vi "Format Script Email.vi"(8 "Script Start/End":enum16{"Start Script", "End Script"}(ring), 9 "Time String":string, 11 "Measurement Information":T1={"Comments"="", "Directory Input"="", "Data file path"=path "C:/Data/EPR Data", "Scripting File"=path "C:/Data/Configuration Script.csv", "Save Data"=FALSE, "Tooth size (d11) [mm]"=0.0, "Tooth size (d12) [mm]"=0.0, "Tooth size (d21) [mm]"=0.0, "Tooth size (d22) [mm]"=0.0, "Dose of Tooth [Gy]"=0.0, "Safe Shutdown?"=FALSE, "Gases Available"=[], "Database Username"="", "Database Password"="", "Database Login URL"="", "Database Upload URL"="", "Database Success URL"="", "Database XML URL"="", "Database Resonator URL"="", "Session Number"=0, "Set #"=0, "Resonator Operator"="", "Session Type"="", "Tooth/Sample ID"="", "Volunteer ID"="", "Computer Operator"="", "Volunteer Type"="", "Site/Tooth Selection (T8,T9)"="", "Resonator"="", "Measurement Site"="", "Non-standard session?"=FALSE, "EPR DAQ Version"="", "Session Path"=path "C:/Data/EPR Data", "Chosen Applied State"="", "Chosen Initial State"="", "Time of Transition"="", "DAQ Mode"=enum."Engineering", "pO2/Scan [mmHg]"=[], "pO2/Set [mmHg]"=[], "Linewidth (HWHM)/Scan [Gauss]"=[], "Linewidth (HWHM)/Set [Gauss]"=[], "pO2 Conversion"="", "Dose Calibration Cluster"={"Dose Response"={"grand_mean"=0.0292016, "slope"=0.0188720543}, "Dose Correction"={"Sex"=1, "a0"=7.719669421, "a1"=-2.746550736, "a2"=-0.186490355, "a3"=0.041922063, "a4"=-0.849147359, "a5"=0.14330063, "a6"=0.019930219, "A_n"=40.0, "H_n"=10.12, "Dose Correction"=FALSE}, "Dose Reporting"={"Reporting is"=TRUE, "sd_threshold [AU]"=0.06, "sd_model [Gy]"=0.66, "dosimetric_threshold [Gy]"=2.0, "Add intrasession errors is"=FALSE, "Prior Radiation?"=FALSE}}, "OxyChip Slope"=0.0, "OxyChip Intercept"=0.0, "QA Mode"=enum."Select QA Mode", "QA Session?"=FALSE, "Sample Type"=enum."Empty Resonator", "Report pO2/Scan"=FALSE, "Skip End Session Save"=FALSE, "Number of sites"=enum."# Probes", "Recipient Name"="", "Sender Name"="", "Recipient Email"="", "Transition State History"=[], "pO2 Report Times"=[], "Temperature [C]"=0.0, "+Error pO2/Scan [mmHg]"=[], "-Error pO2/Scan [mmHg]"=[], "+Error pO2/Set [mmHg]"=[], "-Error pO2/Set [mmHg]"=[], "Oxy Phase Exclusion Tolerance [rad]"=0.0, "Oxy Center Exclusion Tolerance [%]"=0.0, "Oxy Exclude Unacceptable"=FALSE, "Oxy Unacceptable Estimate Flags"=[], "Save Session PPT"=FALSE, "Flagged Bad Sets"=[]} {"Oxy Center Exclusion Tolerance [%]" format="%#_9g"; "Oxy Phase Exclusion Tolerance [rad]" format="%#_9g"; "Temperature [C]" format="%#_9g"; "OxyChip Intercept" format="%#_9g"; "OxyChip Slope" format="%#_9g"; "Dose Calibration Cluster"."Dose Reporting"."dosimetric_threshold [Gy]" format="%#_9g"; "Dose Calibration Cluster"."Dose Reporting"."sd_model [Gy]" format="%#_9g"; "Dose Calibration Cluster"."Dose Reporting"."sd_threshold [AU]" format="%#_9g"; "Dose Calibration Cluster"."Dose Correction"."H_n" format="%#_9g"; "Dose Calibration Cluster"."Dose Correction"."A_n" format="%#_9g"; "Dose Calibration Cluster"."Dose Correction"."a6" format="%#.9g"; "Dose Calibration Cluster"."Dose Correction"."a5" format="%#.9g"; "Dose Calibration Cluster"."Dose Correction"."a4" format="%#.9g"; "Dose Calibration Cluster"."Dose Correction"."a3" format="%#.9g"; "Dose Calibration Cluster"."Dose Correction"."a2" format="%#.9g"; "Dose Calibration Cluster"."Dose Correction"."a1" format="%#.9g"; "Dose Calibration Cluster"."Dose Correction"."a0" format="%#.9g"; "Dose Calibration Cluster"."Dose Correction"."Sex" items=["Male"=1, "Female"=0]; "Dose Calibration Cluster"."Dose Response"."slope" format="%#_9g"; "Dose Calibration Cluster"."Dose Response"."grand_mean" format="%#_9g"}) -> (3 "Measurement Information Out":T1={"Comments"="", "Directory Input"="", "Data file path"=path "C:/Data/EPR Data", "Scripting File"=path "C:/Data/Configuration Script.csv", "Save Data"=FALSE, "Tooth size (d11) [mm]"=0.0, "Tooth size (d12) [mm]"=0.0, "Tooth size (d21) [mm]"=0.0, "Tooth size (d22) [mm]"=0.0, "Dose of Tooth [Gy]"=0.0, "Safe Shutdown?"=FALSE, "Gases Available"=[], "Database Username"="", "Database Password"="", "Database Login URL"="", "Database Upload URL"="", "Database Success URL"="", "Database XML URL"="", "Database Resonator URL"="", "Session Number"=0, "Set #"=0, "Resonator Operator"="", "Session Type"="", "Tooth/Sample ID"="", "Volunteer ID"="", "Computer Operator"="", "Volunteer Type"="", "Site/Tooth Selection (T8,T9)"="", "Resonator"="", "Measurement Site"="", "Non-standard session?"=FALSE, "EPR DAQ Version"="", "Session Path"=path "C:/Data/EPR Data", "Chosen Applied State"="", "Chosen Initial State"="", "Time of Transition"="", "DAQ Mode"=enum."Engineering", "pO2/Scan [mmHg]"=[], "pO2/Set [mmHg]"=[], "Linewidth (HWHM)/Scan [Gauss]"=[], "Linewidth (HWHM)/Set [Gauss]"=[], "pO2 Conversion"="", "Dose Calibration Cluster"={"Dose Response"={"grand_mean"=0.0292016, "slope"=0.0188720543}, "Dose Correction"={"Sex"=1, "a0"=7.719669421, "a1"=-2.746550736, "a2"=-0.186490355, "a3"=0.041922063, "a4"=-0.849147359, "a5"=0.14330063, "a6"=0.019930219, "A_n"=40.0, "H_n"=10.12, "Dose Correction"=FALSE}, "Dose Reporting"={"Reporting is"=TRUE, "sd_threshold [AU]"=0.06, "sd_model [Gy]"=0.66, "dosimetric_threshold [Gy]"=2.0, "Add intrasession errors is"=FALSE, "Prior Radiation?"=FALSE}}, "OxyChip Slope"=0.0, "OxyChip Intercept"=0.0, "QA Mode"=enum."Select QA Mode", "QA Session?"=FALSE, "Sample Type"=enum."Empty Resonator", "Report pO2/Scan"=FALSE, "Skip End Session Save"=FALSE, "Number of sites"=enum."# Probes", "Recipient Name"="", "Sender Name"="", "Recipient Email"="", "Transition State History"=[], "pO2 Report Times"=[], "Temperature [C]"=0.0, "+Error pO2/Scan [mmHg]"=[], "-Error pO2/Scan [mmHg]"=[], "+Error pO2/Set [mmHg]"=[], "-Error pO2/Set [mmHg]"=[], "Oxy Phase Exclusion Tolerance [rad]"=0.0, "Oxy Center Exclusion Tolerance [%]"=0.0, "Oxy Exclude Unacceptable"=FALSE, "Oxy Unacceptable Estimate Flags"=[], "Save Session PPT"=FALSE, "Flagged Bad Sets"=[]} {"Oxy Center Exclusion Tolerance [%]" format="%#_9g"; "Oxy Phase Exclusion Tolerance [rad]" format="%#_9g"; "Temperature [C]" format="%#_9g"; "OxyChip Intercept" format="%#_9g"; "OxyChip Slope" format="%#_9g"; "Dose Calibration Cluster"."Dose Reporting"."dosimetric_threshold [Gy]" format="%#_9g"; "Dose Calibration Cluster"."Dose Reporting"."sd_model [Gy]" format="%#_9g"; "Dose Calibration Cluster"."Dose Reporting"."sd_threshold [AU]" format="%#_9g"; "Dose Calibration Cluster"."Dose Correction"."H_n" format="%#_9g"; "Dose Calibration Cluster"."Dose Correction"."A_n" format="%#_9g"; "Dose Calibration Cluster"."Dose Correction"."a6" format="%#.9g"; "Dose Calibration Cluster"."Dose Correction"."a5" format="%#.9g"; "Dose Calibration Cluster"."Dose Correction"."a4" format="%#.9g"; "Dose Calibration Cluster"."Dose Correction"."a3" format="%#.9g"; "Dose Calibration Cluster"."Dose Correction"."a2" format="%#.9g"; "Dose Calibration Cluster"."Dose Correction"."a1" format="%#.9g"; "Dose Calibration Cluster"."Dose Correction"."a0" format="%#.9g"; "Dose Calibration Cluster"."Dose Correction"."Sex" items=["Male"=1, "Female"=0]; "Dose Calibration Cluster"."Dose Response"."slope" format="%#_9g"; "Dose Calibration Cluster"."Dose Response"."grand_mean" format="%#_9g"})   [LabVIEW 2016]
uses:
  Types/Measurement Information.ctl
  Analysis/Dose Calculation and Reporting/Dose Calculation Control.ctl
  Types/Sample Type.ctl
panel:
  in  "Cancel":bool
  in  "Continue":bool
  in  "Email Address of Recipient":string
  in  "Name of Recipient":string
  in  "Name of Sender":string
  # "Session Information"
  # "Oximetric Data and Information"
  # "Email"
  # "Tooth Information"
  # "Database"
  # "Session Information"
  # "Oximetric Data and Information"
  # "Email"
  # "Tooth Information"
  # "Database"
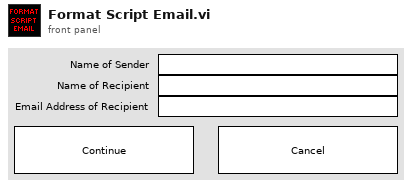
[diagram p1: front panel]
types:
  T1 = typedef "Measurement Information.ctl" = cluster{"Comments":string, "Directory Input":string, "Data file path":path, "Scripting File":path, "Save Data":bool, "Tooth size (d11) [mm]":dbl, "Tooth size (d12) [mm]":dbl, "Tooth size (d21) [mm]":dbl, "Tooth size (d22) [mm]":dbl, "Dose of Tooth [Gy]":dbl, "Safe Shutdown?":bool, "Gases Available":string[], "Database Username":string, "Database Password":string, "Database Login URL":string, "Database Upload URL":string, "Database Success URL":string, "Database XML URL":string, "Database Resonator URL":string, "Session Number":i32, "Set #":u32, "Resonator Operator":string, "Session Type":string, "Tooth/Sample ID":string, "Volunteer ID":string, "Computer Operator":string, "Volunteer Type":string, "Site/Tooth Selection (T8,T9)":string, "Resonator":string, "Measurement Site":string, "Non-standard session?":bool, "EPR DAQ Version":string, "Session Path":path, "Chosen Applied State":string, "Chosen Initial State":string, "Time of Transition":string, "DAQ Mode":enum16{"Engineering", "Dosimetry", "Oximetry"}, "pO2/Scan [mmHg]":dbl[][], "pO2/Set [mmHg]":dbl[][], "Linewidth (HWHM)/Scan [Gauss]":dbl[][], "Linewidth (HWHM)/Set [Gauss]":dbl[][], "pO2 Conversion":string, "Dose Calibration Cluster":T2, "OxyChip Slope":dbl, "OxyChip Intercept":dbl, "QA Mode":enum16{"Select QA Mode", "QA-Start/End", "QA-Mid", "QA-Weekly", "QA-Eng", "Check Calibration"}, "QA Session?":bool, "Sample Type":T3, "Report pO2/Scan":bool, "Skip End Session Save":bool, "Number of sites":enum16{"# Probes", "1", "2", "3", "4"}, "Recipient Name":string, "Sender Name":string, "Recipient Email":string, "Transition State History":string[], "pO2 Report Times":string[], "Temperature [C]":dbl, "+Error pO2/Scan [mmHg]":dbl[][], "-Error pO2/Scan [mmHg]":dbl[][], "+Error pO2/Set [mmHg]":dbl[][], "-Error pO2/Set [mmHg]":dbl[][], "Oxy Phase Exclusion Tolerance [rad]":dbl, "Oxy Center Exclusion Tolerance [%]":dbl, "Oxy Exclude Unacceptable":bool, "Oxy Unacceptable Estimate Flags":bool[], "Save Session PPT":bool, "Flagged Bad Sets":u32[]}
  T2 = typedef "Dose Calculation Control.ctl" = cluster{"Dose Response":cluster{"grand_mean":dbl, "slope":dbl}, "Dose Correction":cluster{"Sex":u16, "a0":dbl, "a1":dbl, "a2":dbl, "a3":dbl, "a4":dbl, "a5":dbl, "a6":dbl, "A_n":dbl, "H_n":dbl, "Dose Correction":bool}, "Dose Reporting":cluster{"Reporting is":bool, "sd_threshold [AU]":dbl, "sd_model [Gy]":dbl, "dosimetric_threshold [Gy]":dbl, "Add intrasession errors is":bool, "Prior Radiation?":bool}}
  T3 = typedef "Sample Type.ctl" = enum16{"Empty Resonator", "IRS", "BallZero", "Irradiated Tooth", "Non-irradiated Tooth", "OxyChip", "LiPc", "PDT", "India Ink"}
  T4 = enum8{"Enabled", "Disabled", "Disabled and Grayed Out"}
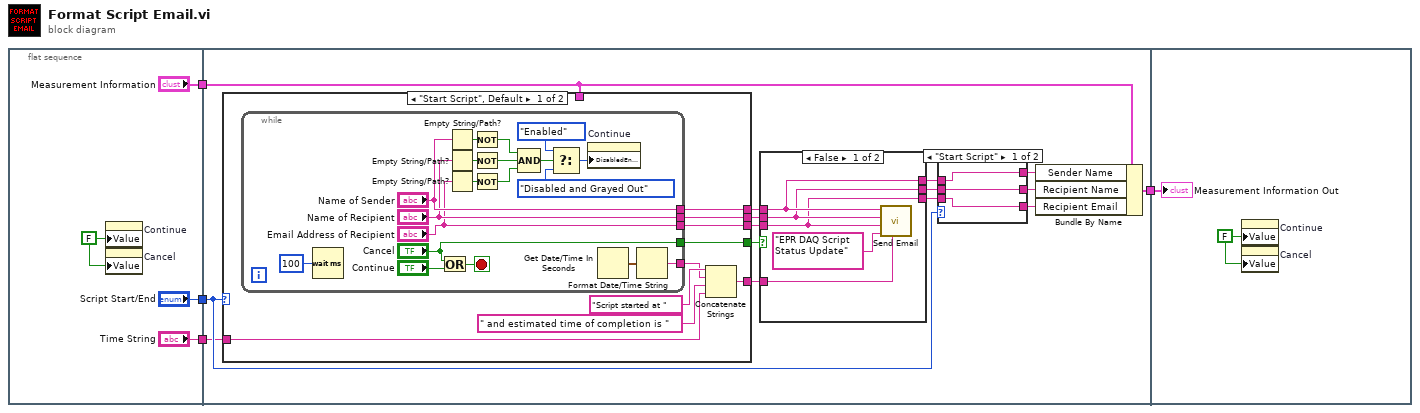
[diagram p0: block diagram]
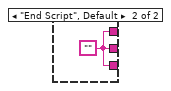
[diagram p2: hidden frame]
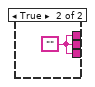
[diagram p3: hidden frame]
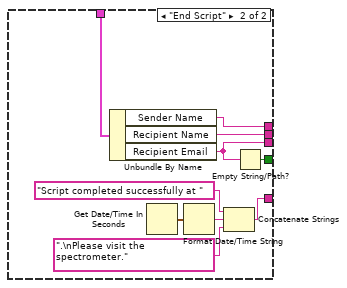
[diagram p4: hidden frame]
diagram:
  n1 = flat-sequence {
    tunnel: ["Script Start/End"] -> w4
    tunnel: ["Time String"] -> w3
    tunnel: ["Measurement Information"] -> w2
    tunnel: w4 -> [w19]
    tunnel: w3 -> [w18]
    tunnel: w2 -> [w13]
    tunnel: [w9] -> w1
    tunnel: w1 -> [w72]
    frame #0 {
      w8 = FALSE ("Continue")
      n2 = property on="Continue" class="Bool (strict)"("Value"=w8) -> ()  [unwired: 2 in, 2 out]
      n3 = property on="Cancel" class="Bool (strict)"("Value"=w8) -> ()  [unwired: 2 in, 2 out]
    }
    frame #1 {
      n4 = case shown="\"Start Script\", Default" w19 {
        tunnel: [w42 w67] -> w23
        tunnel: [w41 w70] -> w22
        tunnel: [w40 w69] -> w21
        tunnel: [w39 w68] -> w20
        tunnel: w18 -> [w36 _]
        tunnel: [w35 w66] -> w17
        tunnel: w13 -> [_ w71]
        frame "Start Script", Default {
          n5 = while {
            tunnel: ["Cancel"] -> w42
            tunnel: ["Name of Sender"] -> w41
            tunnel: ["Name of Recipient"] -> w40
            tunnel: ["Email Address of Recipient"] -> w39
            tunnel: [w43] -> w34
            stop <- w61 stop-if-true
            n6 = Wait (ms)(milliseconds to wait=u32 100) -> ()  [unwired: 1 out]
            n7 = Or(x="Cancel", y="Continue") -> (x .or. y?=w61:bool)
            n8 = Empty String/Path?(string/path="Name of Sender") -> (empty?=w54:bool)
            n9 = Empty String/Path?(string/path="Name of Recipient") -> (empty?=w53:bool)
            n10 = Empty String/Path?(string/path="Email Address of Recipient") -> (empty?=w52:bool)
            n11 = Not(x=w54) -> (.not. x?=w47:bool)
            n12 = Not(x=w53) -> (.not. x?=w46:bool)
            n13 = Not(x=w52) -> (.not. x?=w45:bool)
            n14 = Compound Arithmetic op=AND(w47, w46, w45) -> (w48:bool)
            n15 = Select(t=T4."Enabled" ("Disabled"), s=w48, f=T4."Disabled and Grayed Out" ("Disabled")) -> (s? t:f=w49:T4)
            n16 = property on="Continue" class="Bool (strict)"("DisabledEnum"=w49) -> ()  [unwired: 2 in, 2 out]
            n17 = Get Date/Time In Seconds() -> (seconds since 1Jan1904=w44:timestamp)
            n18 = Format Date/Time String(seconds (now)=w44) -> (date/time string=w43:string)  [unwired: 2 out]
          }
          n19 = Concatenate Strings("Script started at " ("Email Address of Recipient"), w34, " and estimated time of completion is " ("string"), w36) -> (w35:string)
        }
        frame "End Script" {
          n20 = Unbundle By Name(w71) -> ("Sender Name"=w70:string, "Recipient Name"=w69:string, "Recipient Email"=w68:string)
          n21 = Get Date/Time In Seconds() -> (seconds since 1Jan1904=w64:timestamp)
          n22 = Format Date/Time String(seconds (now)=w64) -> (date/time string=w63:string)  [unwired: 2 out]
          n23 = Concatenate Strings("Script completed successfully at " ("Email Address of Recipient"), w63, ".\nPlease visit the spectrometer." ("string")) -> (w66:string)
          n24 = Empty String/Path?(string/path=w68) -> (empty?=w67:bool)
        }
      }
      n25 = case shown="False" w23 {
        tunnel: w22 -> [w30 _]
        tunnel: w21 -> [w29 _]
        tunnel: w20 -> [w28 _]
        tunnel: w17 -> [w31 _]
        tunnel: [w30 w33] -> w16
        tunnel: [w29 w33] -> w15
        tunnel: [w28 w33] -> w14
        frame False {
          n26 = call "Send Email.vi"("Sender's Name"=w30, "Recipient's Name"=w29, "Recipient's Email Address Address"=w28, "Subject"="EPR DAQ Script Status Update", "Body"=w31) -> ()  [unwired: 2 in]
        }
        frame True {
          w33 = ""
        }
      }
      n27 = case shown="\"Start Script\"" w19 {
        tunnel: w16 -> [w26 _]
        tunnel: w15 -> [w25 _]
        tunnel: w14 -> [w24 _]
        tunnel: [w26 w27] -> w12
        tunnel: [w25 w27] -> w11
        tunnel: [w24 w27] -> w10
        frame "Start Script" {
        }
        frame "End Script", Default {
          w27 = ""
        }
      }
      n28 = Bundle By Name(cluster=w13, "Sender Name"=w12, "Recipient Name"=w11, "Recipient Email"=w10) -> (w9:T1)
    }
    frame #2 {
      w73 = FALSE ("Continue")
      n29 = property on="Continue" class="Bool (strict)"("Value"=w73) -> ()  [unwired: 2 in, 2 out]
      n30 = property on="Cancel" class="Bool (strict)"("Value"=w73) -> ()  [unwired: 2 in, 2 out]
      "Measurement Information Out" <- w72
    }
  }
